vi "Untitled dd 4.vi"(8 "error in":errorcluster, 11 "Class 4 in":refnum<class "Class 4.lvclass">) -> (0 "error out":errorcluster, 3 "Class 4 out":refnum<class "Class 4.lvclass">)   [LabVIEW 2020, in "Class 4.lvclass"]
uses:
  Class 4.lvclass
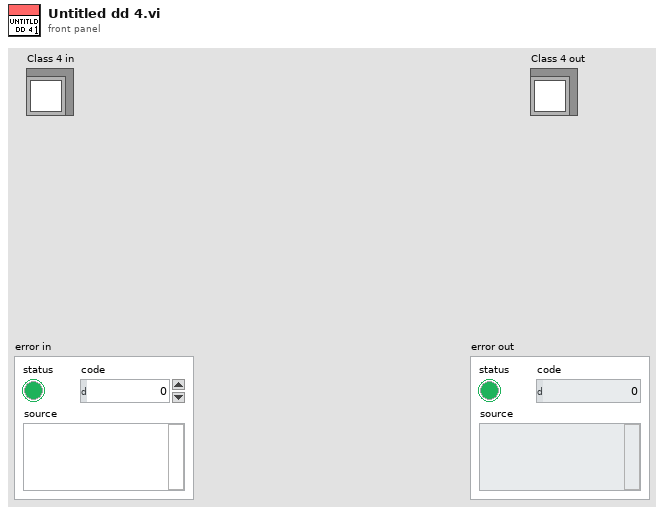
[diagram p1: front panel]
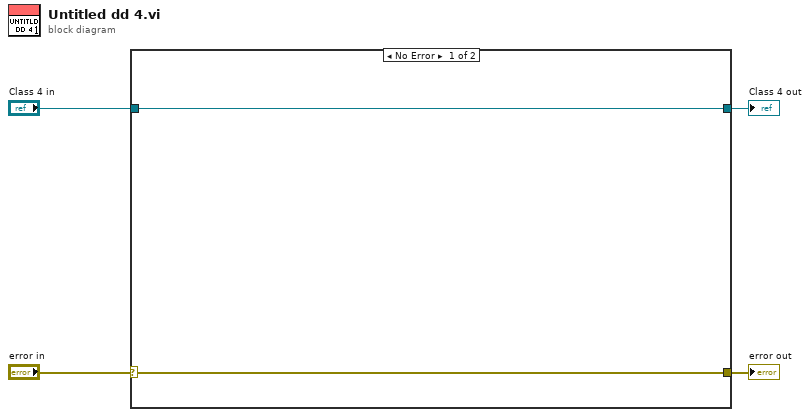
[diagram p0: block diagram]
diagram:
  n1 = case shown="No Error" "error in" {
    selector: "error in" -> [w5 w8]
    tunnel: [w5 w8] -> w1
    tunnel: [w6 w7] -> w3
    tunnel: "Class 4 in" -> [w6 w7]
    frame No Error {
    }
    frame Error {
    }
  }
  "Class 4 out" <- w3
  "error out" <- w1
